vi "RMCreate.vi"(6 "Frame info names":string[](array[string]), 8 "frame info file":path, 9 "output file":path, 10 "ResultManagerConfig":T2) -> (3 "ResultManager":T1)   [LabVIEW 2011]
doc: "Create a result manager instance. The output files and configuration are passed through this method, but the tracker that is being checked for new results still has to be set with RMSetTracker.vi"
uses:
  ResultManagerConfig.ctl
  XYZf.ctl
  ResultManagerInstance.ctl
  QTrkDLL.vi
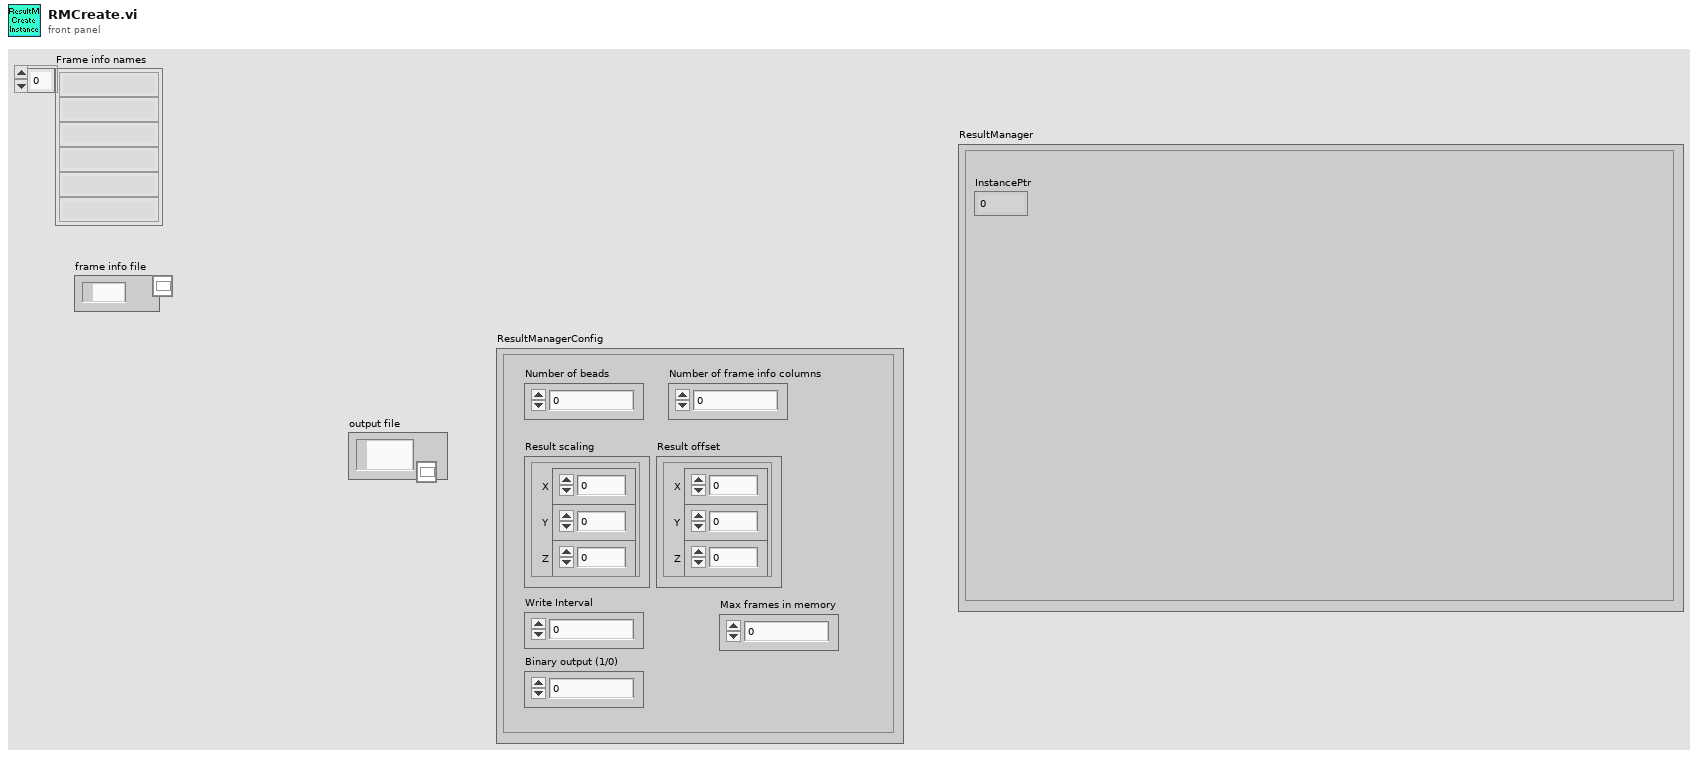
[diagram p1: front panel]
types:
  T1 = typedef "ResultManagerInstance.ctl" = cluster{"InstancePtr":u64}
  T2 = typedef "ResultManagerConfig.ctl" = cluster{"Number of beads":i32, "Number of frame info columns":i32, "Result scaling":T3, "Result offset":T3, "Write Interval":i32, "Max frames in memory":i32, "Binary output (1/0)":i8}
  T3 = typedef "XYZf.ctl" = cluster{"X":sgl, "Y":sgl, "Z":sgl}
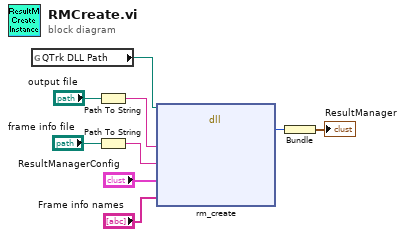
[diagram p0: block diagram]
diagram:
  n1 = global read "QTrkDLL.vi" "QTrk DLL Path"() -> (w9:path)
  n2 = Path To String(path="output file") -> (string=w6:string)
  n3 = Path To String(path="frame info file") -> (string=w4:string)
  n4 = dll-call lib="D:/jcnossen1/cudaqi-tracker/bin/jtrk-labview.dll" fn="rm_create"(path in=w9, "file"=w6, "frameInfoFile"=w4, "config"="ResultManagerConfig", "frameInfoColNames"="Frame info names") -> ("result manager ptr"=w2:u64)  [unwired: 6 in, 2 out]
  n5 = Bundle("result manager ptr"=w2) -> (→"ResultManager":cluster{"result manager ptr":u64})  [unwired: 1 in]
